vi "test Loopback_Acyclic_withOverflow.vi"(8 "error in":errorcluster, 11 "TestCase in":refnum<class "SingleCore.lvclass">) -> (0 "error out":errorcluster, 3 "TestCase out":refnum<class "SingleCore.lvclass">)   [LabVIEW 2020, in "SingleCore.lvclass"]
uses:
  SingleCore.lvclass
  C:/Git/niveristand-custom-device-testing-tools/VeriStandTestCase/VeriStandTestCase.lvclass
  4b06c685-66bb-4135-9ad1-d89a50a95502.vi
  <vilib>/numeric/Random Number (Range) I64.vi
  <vilib>/numeric/sub_Random U32.vi
  <vilib>/NI VeriStand/Execution/Workspace/NI VeriStand - Set Multiple Channel Values.vi
  <vilib>/NI VeriStand/Execution/Workspace/NI VeriStand - Set Single Channel Value.vi
  <vilib>/NI VeriStand/Execution/Workspace/NI VeriStand - Get Single Channel Value.vi
  <vilib>/addons/_JKI Toolkits/VI Tester/TestCase.llb/TestCase.lvclass
  <vilib>/NI VeriStand/Execution/Workspace/NI_VS Workspace ExecutionAPI.lvlib
  C:/Program Files (x86)/National Instruments/LabVIEW 2020/vi.lib/addons/_JKI Toolkits/VI Tester/TestCase.llb/TestCase.lvclass
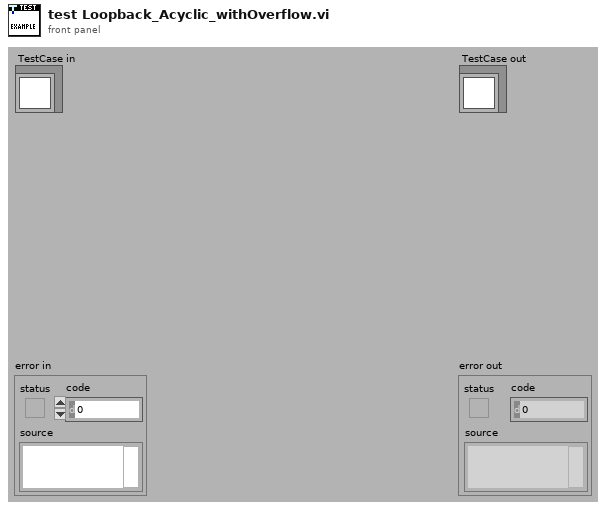
[diagram p1: front panel]
types:
  T1 = typedef "NI_VS Workspace ExecutionAPI.lvlib/WorkspaceAPI.ctl" = refnum<k24>
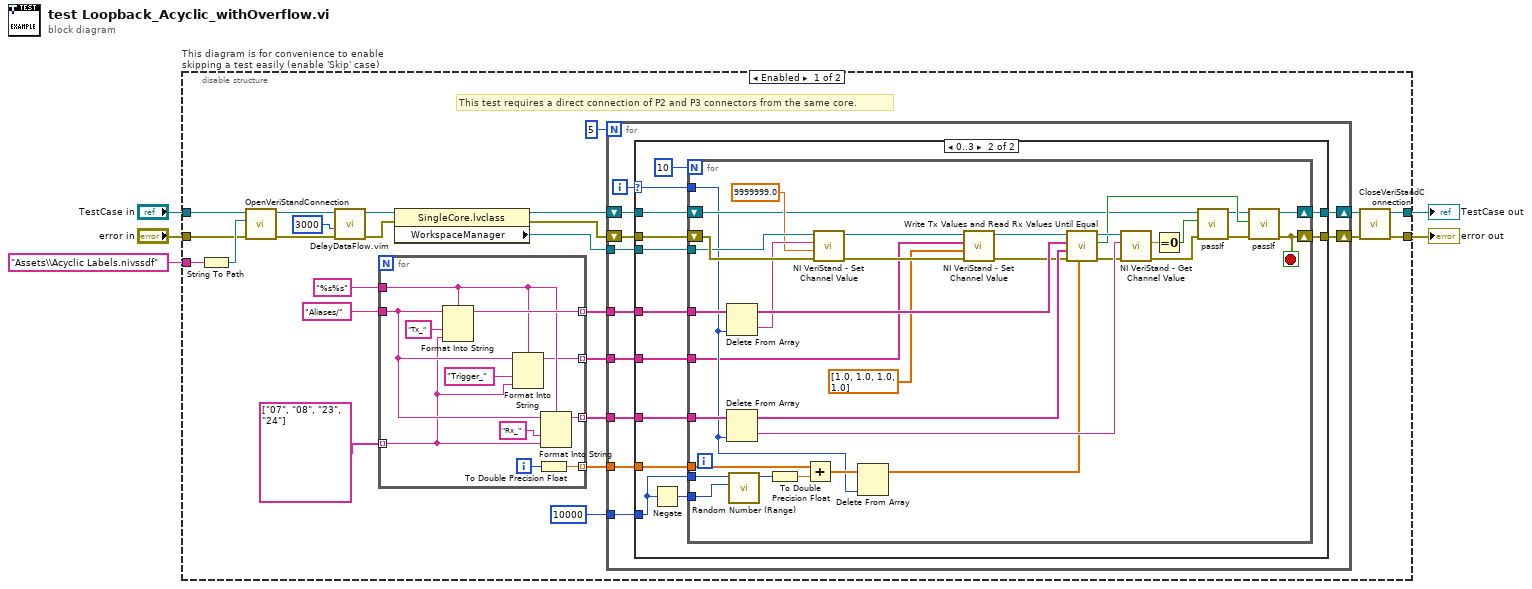
[diagram p0: block diagram]
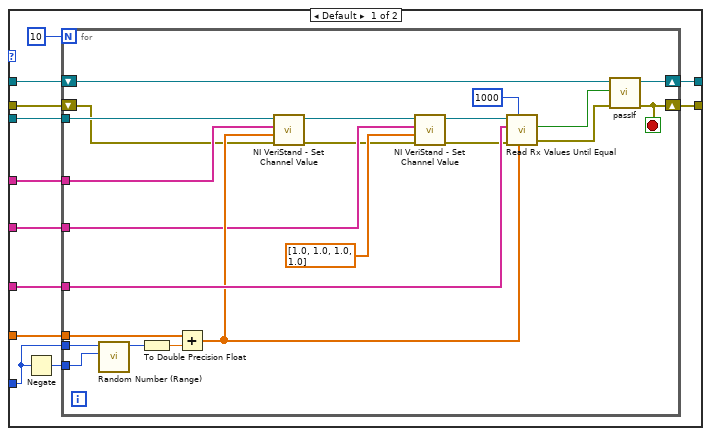
[diagram p2: hidden frame]
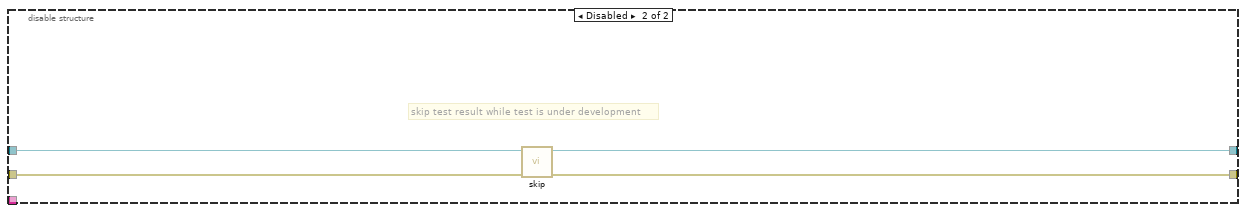
[diagram p3: hidden frame]
diagram:
  n1 = disable-structure "This diagram is for convenience to enable skipping a test easily (enable 'Skip' case)" shown="Enabled" {
    disable-tunnel: "TestCase in" -> [w24 w136]
    disable-tunnel: [w21 w134] -> w2
    disable-tunnel: [w20 w135] -> w4
    disable-tunnel: "error in" -> [w23 w133]
    disable-tunnel: "Assets\\Acyclic Labels.nivssdf" ("Channel") -> [w22 _]
    frame Enabled {
      # "This test requires a direct connection of P2 and P3 connectors from the same core."
      n2 = String To Path(string=w22) -> (path=w25:path)
      n3 = call-dynamic "OpenVeriStandConnection.vi"("error in (no error)"=w23, "System Definition File"=w25, "VeriStand Test Case in"=w24) -> ("error out"=w27:errorcluster, "VeriStand Test Case out"=w29:refnum<class "SingleCore.lvclass">)  [unwired: 6 in, 1 out]
      n4 = call "DelayDataFlow.vim"("value in"=w27, "milliseconds to wait"=u32 3000) -> ("value out"=w26:errorcluster)  [unwired: 2 in, 1 out]
      n5 = for {
        tunnel: [w132] -> w17 mode=indexing
        tunnel: [w127] -> w14 mode=indexing
        tunnel: [w131] -> w19 mode=indexing
        tunnel: "Aliases/" ("Channel") -> [w125]
        tunnel: string[] ["07", "08", "23", "24"] -> [w123] mode=indexing
        tunnel: "%s%s" ("format string") -> [w126]
        tunnel: [w122] -> w6 mode=indexing
        i -> [w130]
        n6 = Format Into String(format string=w126, initial string=w125, "Tx_" ("input 1"), w123) -> (resulting string=w132:string)  [unwired: 1 in, 1 out]
        n7 = Format Into String(format string=w126, initial string=w125, "Trigger_" ("input 1"), w123) -> (resulting string=w122:string)  [unwired: 1 in, 1 out]
        n8 = To Double Precision Float(number=w130) -> (double precision float=w131:dbl)
        n9 = Format Into String(format string=w126, initial string=w125, "Rx_" ("input 1"), w123) -> (resulting string=w127:string)  [unwired: 1 in, 1 out]
      }
      n10 = property class="SingleCore.lvclass"(reference=w29, error in=w26) -> (reference out=w13:refnum<class "SingleCore.lvclass">, error out=w15:errorcluster, "WorkspaceManager"=w16:T1)
      n11 = for {
        N: 5 -> [_]
        tunnel: w19 -> [w40]
        tunnel: i64 10000 ("upper bound (100)") -> [w39]
        tunnel: w17 -> [w38]
        tunnel: w16 -> [w37]
        tunnel: w14 -> [w35]
        shift-right: [w32] -> w11
        shift-left: w15 -> [w36]
        shift-right: [w33] -> w12
        shift-left: w13 -> [w34]
        tunnel: w6 -> [w30]
        i -> [w31]
        n12 = case shown="0..3" w31 {
          selector: w31 -> [_ w76]
          tunnel: w40 -> [w52 w87]
          tunnel: w39 -> [w51 w86]
          tunnel: w38 -> [w49 w84]
          tunnel: w37 -> [w48 w83]
          tunnel: w36 -> [w47 w82]
          tunnel: w35 -> [w46 w81]
          tunnel: w34 -> [w45 w80]
          tunnel: [w44 w79] -> w33
          tunnel: [w43 w78] -> w32
          tunnel: w30 -> [w41 w75]
          frame Default {
            n13 = Negate(x=w51) -> (-x=w50:i64)
            n14 = for {
              N: 10 -> [_]
              tunnel: w52 -> [w72]
              tunnel: w51 -> [w71]
              tunnel: w50 -> [w70]
              tunnel: w49 -> [w69]
              tunnel: w48 -> [w58]
              tunnel: w46 -> [w68]
              shift-right: [w65] -> w44
              shift-left: w45 -> [w66]
              shift-right: [w63] -> w43
              shift-left: w47 -> [w53]
              tunnel: w41 -> [w60]
              stop <- w63 stop-if-true
              n15 = call-poly <vilib>:"Random Number (Range).vi"("lower bound (-100)"=w70, "upper bound (100)"=w71) -> ("number"=w74:i64)  [unwired: 9 in]
              n16 = To Double Precision Float(number=w74) -> (double precision float=w73:dbl)
              n17 = Add(x=w72, y=w73) -> (x+y=w64:dbl[])
              n18 = call-poly <vilib>:"NI VeriStand - Set Channel Value.vi"("error in (no error)"=w53, "Values"=w64, "Channels"=w69, "WorkspaceManager in"=w58) -> ("error out"=w54:errorcluster, "WorkspaceManager out"=w57:T1)  [unwired: 6 in]
              n19 = call-poly <vilib>:"NI VeriStand - Set Channel Value.vi"("error in (no error)"=w54, "Values"=dbl[] [1.0, 1.0, 1.0, 1.0], "Channels"=w60, "WorkspaceManager in"=w57) -> ("error out"=w55:errorcluster, "WorkspaceManager out"=w56:T1)  [unwired: 6 in]
              n20 = call "Read Rx Values Until Equal.vi"("expected values"=w64, "timeout (1000 ms)"=1000, "error in"=w55, "Rx aliases"=w68, "workspace manager in"=w56) -> ("error out"=w67:errorcluster, "values equal expected"=w62:bool)  [unwired: 4 in, 1 out]
              n21 = call-dynamic "passIf.vi"("error in (no error)"=w67, "pass"=w62, "TestCase in"=w66) -> ("error out"=w63:errorcluster, "TestCase out"=w65:refnum<class "SingleCore.lvclass">)  [unwired: 7 in]
            }
          }
          frame 0..3 {
            n22 = Negate(x=w86) -> (-x=w85:i64)
            n23 = for {
              N: 10 -> [_]
              tunnel: w87 -> [w119]
              tunnel: w86 -> [w118]
              tunnel: w85 -> [w117]
              tunnel: w84 -> [w113]
              tunnel: w83 -> [w109]
              tunnel: w81 -> [w111]
              shift-right: [w116] -> w79
              shift-left: w80 -> [w101]
              shift-right: [w115] -> w78
              shift-left: w82 -> [w110]
              tunnel: w76 -> [w95]
              tunnel: w75 -> [w89]
              stop <- w115 stop-if-true
              n24 = Delete From Array(array=w113, index=w95) -> (deleted portion=w108:string, array with subset deleted=w114:string[])  [unwired: 1 in]
              n25 = Delete From Array(array=w111, index=w95) -> (deleted portion=w106:string, array with subset deleted=w112:string[])  [unwired: 1 in]
              n26 = call-poly <vilib>:"Random Number (Range).vi"("lower bound (-100)"=w117, "upper bound (100)"=w118) -> ("number"=w121:i64)  [unwired: 9 in]
              n27 = To Double Precision Float(number=w121) -> (double precision float=w120:dbl)
              n28 = Add(x=w119, y=w120) -> (x+y=w96:dbl[])
              n29 = call-poly <vilib>:"NI VeriStand - Set Channel Value.vi"("error in (no error)"=w110, "Value"=9999999.0, "Channel"=w108, "WorkspaceManager in"=w109) -> ("error out"=w93:errorcluster, "WorkspaceManager out"=w92:T1)  [unwired: 6 in]
              n30 = Delete From Array(array=w96, index=w95) -> (array with subset deleted=w94:dbl[])  [unwired: 1 in, 1 out]
              n31 = call-poly <vilib>:"NI VeriStand - Set Channel Value.vi"("error in (no error)"=w93, "Values"=dbl[] [1.0, 1.0, 1.0, 1.0], "Channels"=w89, "WorkspaceManager in"=w92) -> ("error out"=w90:errorcluster, "WorkspaceManager out"=w91:T1)  [unwired: 6 in]
              n32 = call "Write Tx Values and Read Rx Values Until Equal.vi"("Tx values"=w94, "error in"=w90, "Rx aliases"=w112, "Tx aliases"=w114, "workspace manager in"=w91) -> ("error out"=w104:errorcluster, "values equal"=w102:bool, "workspace manager out"=w105:T1)  [unwired: 4 in]
              n33 = call-poly <vilib>:"NI VeriStand - Get Channel Value.vi"("error in (no error)"=w104, "Channel"=w106, "WorkspaceManager in"=w105) -> ("error out"=w100:errorcluster, "Value"=w103:dbl)  [unwired: 6 in, 1 out]
              n34 = Equal To 0?(x=w103) -> (x = 0?=w97:bool)
              n35 = call-dynamic "passIf.vi"("error in (no error)"=w100, "pass"=w97, "TestCase in"=w101) -> ("error out"=w99:errorcluster, "TestCase out"=w98:refnum<class "SingleCore.lvclass">)  [unwired: 7 in]
              n36 = call-dynamic "passIf.vi"("error in (no error)"=w99, "pass"=w102, "TestCase in"=w98) -> ("error out"=w115:errorcluster, "TestCase out"=w116:refnum<class "SingleCore.lvclass">)  [unwired: 7 in]
            }
          }
        }
      }
      n37 = call-dynamic "CloseVeriStandConnection.vi"("error in (no error)"=w11, "VeriStand Test Case in"=w12) -> ("error out"=w20:errorcluster, "VeriStand Test Case out"=w21:refnum<class "SingleCore.lvclass">)  [unwired: 8 in]
    }
    frame Disabled {
      # "skip test result while test is under development"
      n38 = call <vilib>:"skip.vi"("error in (no error)"=w133, "TestCase in"=w136) -> ("error out"=w135:errorcluster, "TestCase out"=w134:refnum<class "SingleCore.lvclass">)  [unwired: 8 in]
    }
  }
  "error out" <- w4
  "TestCase out" <- w2
